vi "Write port.vi"(8 "error in (no error)":errorcluster, 10 "port":u16, 11 "ESP301viaTCPIP in":refnum<class "ESP301viaTCPIP.lvclass">) -> (0 "error out":errorcluster, 3 "ESP301viaTCPIP out":refnum<class "ESP301viaTCPIP.lvclass">)   [LabVIEW 2019, in "ESP301viaTCPIP.lvlib" / "ESP301viaTCPIP.lvclass"]
uses:
  ESP301viaTCPIP.lvclass
  ESP301viaTCPIP.lvclass/ESP301viaTCPIP.ctl
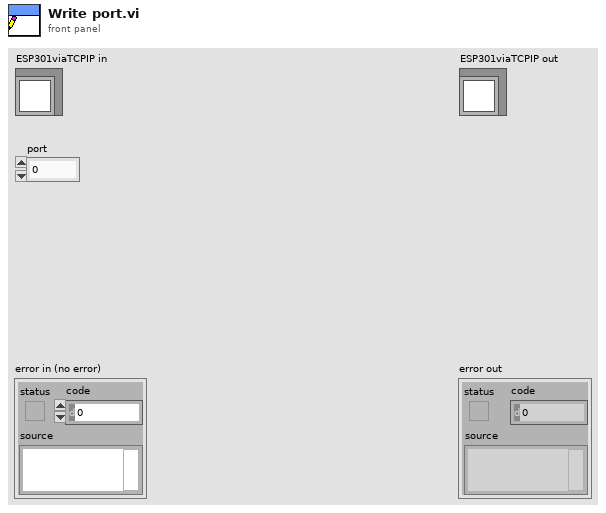
[diagram p1: front panel]
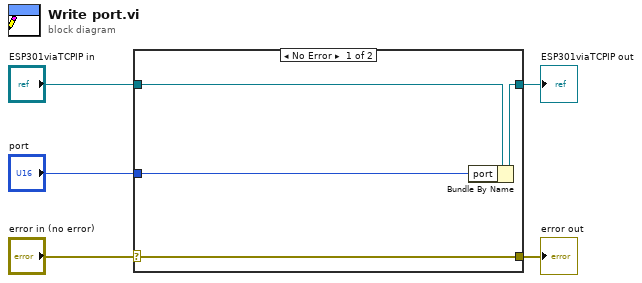
[diagram p0: block diagram]
diagram:
  n1 = case shown="No Error" "error in (no error)" {
    selector: "error in (no error)" -> [w9 w10]
    tunnel: [w9 w10] -> w4
    tunnel: [w7 w11] -> w2
    tunnel: "ESP301viaTCPIP in" -> [w8 w11]
    tunnel: "port" -> [w6 _]
    frame No Error {
      n2 = Bundle By Name(cluster=w8, "port"=w6) -> (w7:refnum<class "ESP301viaTCPIP.lvclass">)
    }
    frame Error {
    }
  }
  "error out" <- w4
  "ESP301viaTCPIP out" <- w2
